vi "averaging_filter.vi"(6 "Reset":bool, 8 "Order":i32, 9 "Time constant (samples)":dbl, 11 "Input":dbl[](array[numeric])) -> (0 "Order variance":dbl[](array[numeric]), 1 "Order mean":dbl[](array[numeric]), 2 "Variance":dbl[](array[numeric]), 3 "Mean":dbl[](array[numeric]))   [LabVIEW 2014]
panel:
  in  "Weights":dbl[](array[numeric])
  # "Filter first-order time constant"
  # "Repeat period.  Changing order causes filter to reset."
  # "\"Order ...\" outputs are contents of the internal  buffers, with length \"Order\".   These are synchronous with the repeat period."
  # "Ignore input contents, but advance filter position."
  # "Reset clears state to zeroes.  Filter must then settle to the steady-state output (multiple time constants)."
  # "Mean and variance of a repeating signal with known repeat period (order).  Input may be any length; mean and variance outputs are the same size as input.  This is like the averaging function on an oscilliscope.  As long as the time constant is much longer than the filter order, only signals that are synchronous with the order pass through into the mean.   In the frequency domain, we pass the order and harmonics of it. \n\nVariance is the filtered mean-squared difference between the input and the mean. This represents the expected variation at each position in the repeat period."
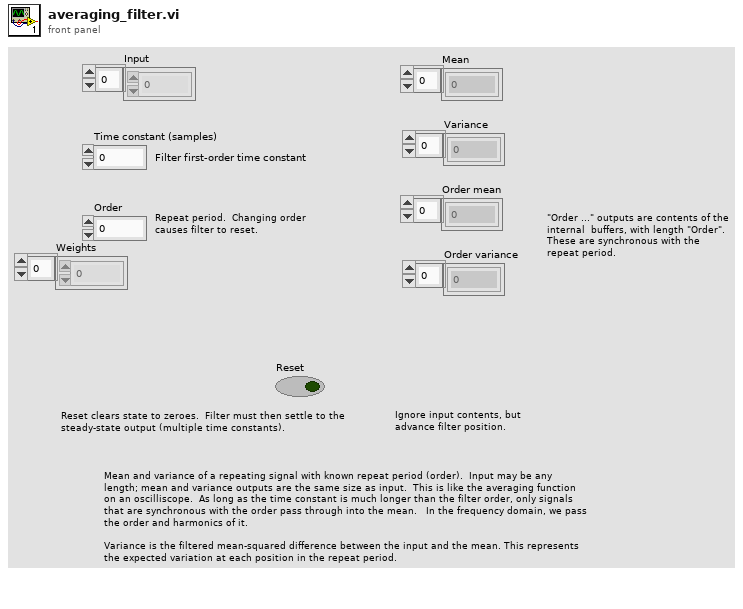
[diagram p1: front panel]
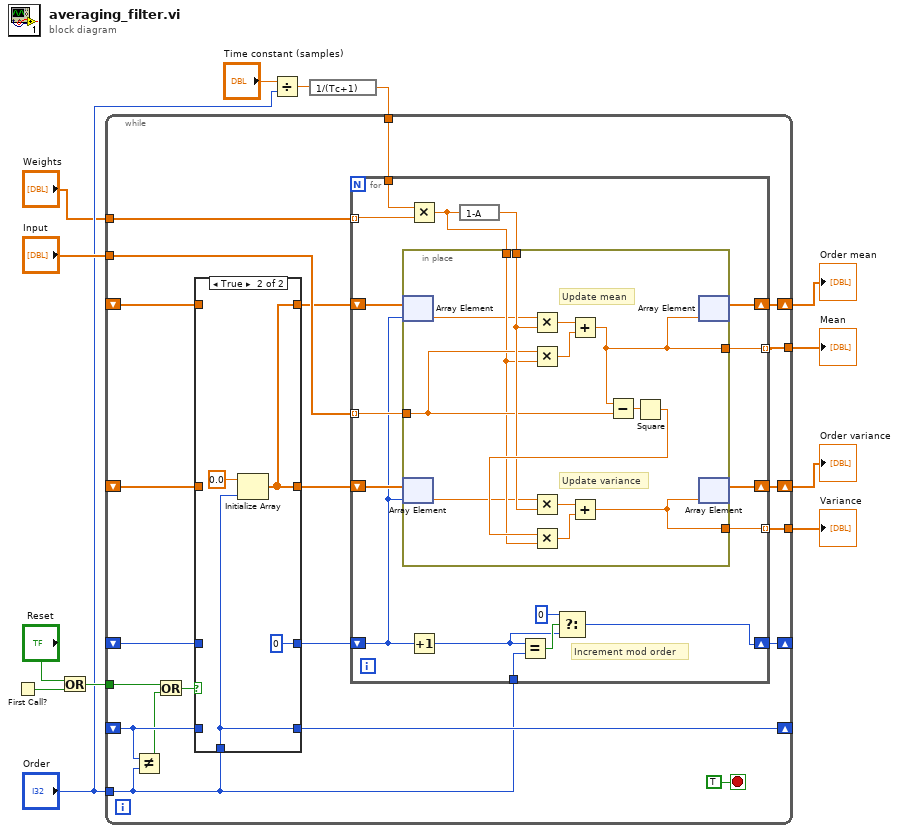
[diagram p0: block diagram]
diagram:
  n1 = First Call?() -> (First Call?: T/F=w10:bool)
  n2 = Or(x="Reset", y=w10) -> (x .or. y?=w8:bool)
  n3 = Divide(x="Time constant (samples)", y="Order") -> (x/y=w7:dbl)
  n4 = expression code="1/(Tc+1)"(w7) -> (w4:dbl)
  n5 = while {
    shift-right: [w26] -> w2
    shift-left: _ -> [w33]
    shift-right: [w27] -> w3
    shift-left: _ -> [w32]
    tunnel: w8 -> [w20]
    tunnel: "Order" -> [w18]
    shift-right: [w22] -> _
    shift-left: _ -> [w31]
    tunnel: "Input" -> [w30]
    tunnel: [w24] -> w12
    tunnel: [w23] -> w11
    tunnel: w4 -> [w15]
    shift-right: [w21] -> _
    shift-left: _ -> [w19]
    tunnel: "Weights" -> [w14]
    stop <- TRUE stop-if-true
    n6 = Not Equal?(x=w19, y=w18) -> (x != y?=w17:bool)
    n7 = Or(x=w20, y=w17) -> (x .or. y?=w16:bool)
    n8 = case shown="True" w16 {
      tunnel: w18 -> [_ w69]
      tunnel: w33 -> [w68 _]
      tunnel: [w68 w71] -> w28
      tunnel: [w67 w71] -> w29
      tunnel: w32 -> [w67 _]
      tunnel: [w66 0 ("Order")] -> w25
      tunnel: w31 -> [w66 _]
      tunnel: w19 -> [w65 _]
      tunnel: [w65 w69] -> w21
      frame False {
      }
      frame True {
        n9 = Initialize Array(0.0 ("Decay"), w69) -> (w71:dbl[])
      }
    }
    n10 = for {
      tunnel: w30 -> [w51] mode=indexing
      shift-right: [w42] -> w22
      shift-left: w25 -> [w47]
      tunnel: w18 -> [w45]
      tunnel: [w41] -> w23 mode=indexing
      tunnel: [w40] -> w24 mode=indexing
      shift-right: [w39] -> w26
      shift-left: w28 -> [w48]
      shift-right: [w49] -> w27
      shift-left: w29 -> [w50]
      tunnel: w15 -> [w37]
      tunnel: w14 -> [w36] mode=indexing
      # "Increment mod order"
      n11 = Multiply(x=w37, y=w36) -> (x*y=w35:dbl)
      n12 = Increment(x=w47) -> (x+1=w44:i32)
      n13 = expression code="1-A"(w35) -> (w38:dbl)
      n14 = in-place {
        in-place-border: w38 -> [w63]
        in-place-border: w51 -> [w57]
        in-place-border: w35 -> [w56]
        in-place-border: [w53] -> w41
        in-place-border: [w52] -> w40
        # "Update variance"
        # "Update mean"
        n15 = in-place-array #1(w50, w47) -> (w55:dbl)
        n16 = in-place-array #2(w48, w47) -> (w54:dbl)
        n17 = Multiply(x=w55, y=w63) -> (x*y=w58:dbl)
        n18 = Multiply(x=w57, y=w56) -> (x*y=w59:dbl)
        n19 = Multiply(x=w54, y=w63) -> (x*y=w62:dbl)
        n20 = Add(x=w58, y=w59) -> (x+y=w53:dbl)
        n21 = Subtract(x=w53, y=w57) -> (x-y=w60:dbl)
        n22 = Square(x=w60) -> (x^2=w64:dbl)
        n23 = Multiply(x=w64, y=w56) -> (x*y=w61:dbl)
        n24 = Add(x=w62, y=w61) -> (x+y=w52:dbl)
        n25 = in-place-array #1(w53) -> (w49:dbl[])  [unwired: 1 out]
        n26 = in-place-array #2(w52) -> (w39:dbl[])  [unwired: 1 out]
      }
      n27 = Equal?(x=w44, y=w45) -> (x = y?=w46:bool)
      n28 = Select(t=0, s=w46, f=w44) -> (s? t:f=w42:i32)
    }
  }
  "Mean" <- w11
  "Variance" <- w12
  "Order mean" <- w3
  "Order variance" <- w2
